vi "get_info.vi"(0 "HGF_ThreadPool":refnum<class "HGF_ThreadPool.lvclass">, 5 "error in (no error)":errorcluster) -> (9 "nofTasksInQueueOut":i32, 11 "nofTasksWaiting":i32, 12 "incThreads":i32, 13 "autoIncrementLimit":i32=-1, 14 "dup HGF_ThreadPool":refnum<class "HGF_ThreadPool.lvclass">, 15 "initialNofThreads":i32, 16 "nofThreads":i32, 17 "maxNofThreads":i32, 18 "HGF_ThreadWorker":refnum<class "HGF_ThreadWorker.lvclass">, 19 "error out":errorcluster)   [LabVIEW 2014, in "HGF_BaseClasses.lvlib" / "HGF_ThreadPool.lvclass"]
doc: "This VI returns some ThreadPool information."
uses:
  HGF_ThreadPool.lvclass
  HGF_ThreadWorker/HGF_ThreadWorker.lvclass
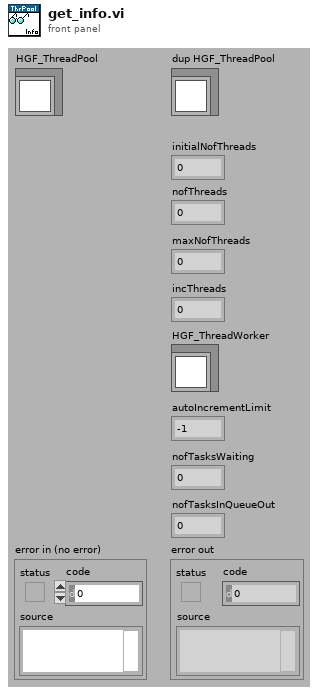
[diagram p1: front panel]
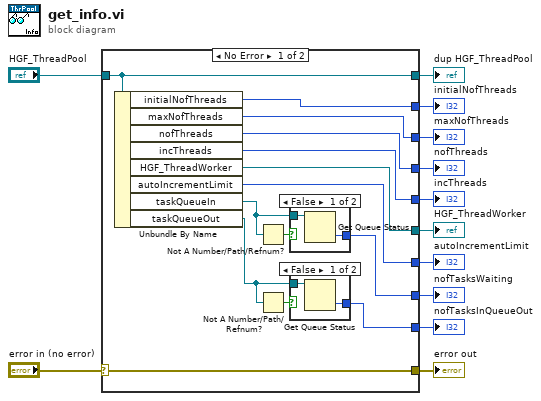
[diagram p0: block diagram]
diagram:
  n1 = case shown="No Error" "error in (no error)" {
    selector: "error in (no error)" -> [w26 w31]
    tunnel: [w26 w31] -> w11
    tunnel: [w25 w32] -> w9
    tunnel: "HGF_ThreadPool" -> [w25 w32]
    tunnel: [w24 _] -> w8
    tunnel: [w23 _] -> w7
    tunnel: [w22 _] -> w6
    tunnel: [w21 _] -> w5
    tunnel: [w20 _] -> w4
    tunnel: [w19 _] -> w3
    tunnel: [w18 _] -> w2
    tunnel: [w13 _] -> w1
    frame No Error {
      n2 = Unbundle By Name(w25) -> ("initialNofThreads"=w24:i32, "maxNofThreads"=w23:i32, "nofThreads"=w22:i32, "incThreads"=w21:i32, "HGF_ThreadWorker"=w20:refnum<class "HGF_ThreadWorker.lvclass">, "autoIncrementLimit"=w19:i32, "taskQueueIn"=w17:refnum<queue>, "taskQueueOut"=w14:refnum<queue>)
      n3 = Not A Number/Path/Refnum?(number/path/refnum=w17) -> (NaN/Path/Refnum?=w16:bool)
      n4 = Not A Number/Path/Refnum?(number/path/refnum=w14) -> (NaN/Path/Refnum?=w15:bool)
      n5 = case shown="False" w16 {
        tunnel: [w30 _] -> w18
        tunnel: w17 -> [w29 _]
        frame False {
          n6 = Get Queue Status(queue=w29) -> (# elements in queue=w30:i32)  [unwired: 1 in, 8 out]
        }
        frame True {
        }
      }
      n7 = case shown="False" w15 {
        tunnel: [w28 _] -> w13
        tunnel: w14 -> [w27 _]
        frame False {
          n8 = Get Queue Status(queue=w27) -> (# elements in queue=w28:i32)  [unwired: 1 in, 8 out]
        }
        frame True {
        }
      }
    }
    frame Error {
    }
  }
  "error out" <- w11
  "dup HGF_ThreadPool" <- w9
  "initialNofThreads" <- w8
  "HGF_ThreadWorker" <- w4
  "maxNofThreads" <- w7
  "nofThreads" <- w6
  "incThreads" <- w5
  "autoIncrementLimit" <- w3
  "nofTasksWaiting" <- w2
  "nofTasksInQueueOut" <- w1
